vi "Convert Attributes to Name-Value Pairs with Type.vi"(11 "JSON Attributes":string) -> (3 "Name-Value Pairs":T1[](array[typedef]))   [LabVIEW 2015, in "NI_JSON Parsing.lvlib"]
uses:
  NI_JSON Parsing.lvlib
  Name-Value with Type.ctl
  Name Value Pair.ctl
  JSON Type.ctl
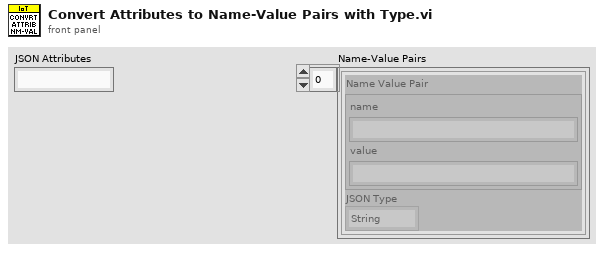
[diagram p1: front panel]
types:
  T1 = typedef "NI_JSON Parsing.lvlib/Name-Value with Type.ctl" = cluster{"Name Value Pair":T2, "JSON Type":T3}
  T2 = typedef "NI_JSON Parsing.lvlib/Name Value Pair.ctl" = cluster{"name":string, "value":string}
  T3 = typedef "NI_JSON Parsing.lvlib/JSON Type.ctl" = enum16{"String", "Numeric", "Boolean"}
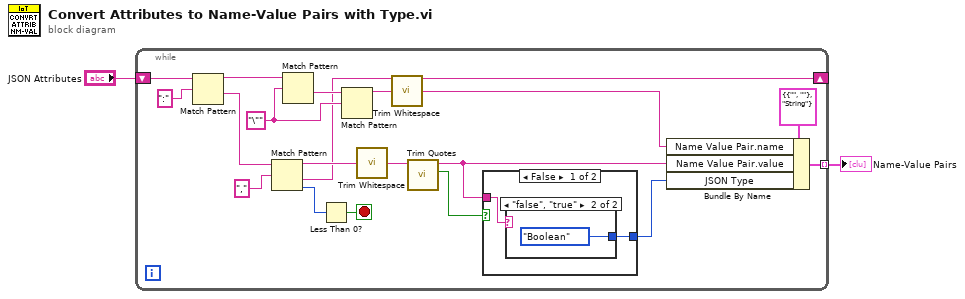
[diagram p0: block diagram]
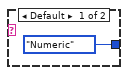
[diagram p2: hidden frame]
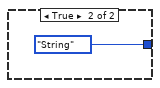
[diagram p3: hidden frame]
diagram:
  n1 = while {
    shift-right: [w10] -> _
    shift-left: "JSON Attributes" -> [w21]
    tunnel: [w8] -> w2 mode=indexing
    stop <- w12 stop-if-true
    w17 = "\"" ("regular expression")
    n2 = Match Pattern(string=w21, regular expression=":") -> (before substring=w19:string, after substring=w15:string)  [unwired: 1 in, 2 out]
    n3 = Match Pattern(string=w15, regular expression=",") -> (before substring=w11:string, after substring=w10:string, offset past match=w13:i32)  [unwired: 1 in, 1 out]
    n4 = Match Pattern(string=w19, regular expression=w17) -> (after substring=w18:string)  [unwired: 1 in, 3 out]
    n5 = Less Than 0?(x=w13) -> (x < 0?=w12:bool)
    n6 = Match Pattern(string=w18, regular expression=w17) -> (before substring=w16:string)  [unwired: 1 in, 3 out]
    n7 = call <vilib>:"Trim Whitespace.vi"("string"=w11) -> ("trimmed string"=w6:string)  [unwired: 1 in]
    n8 = call <vilib>:"Trim Whitespace.vi"("string"=w16) -> ("trimmed string"=w7:string)  [unwired: 1 in]
    n9 = call "Trim Quotes.vi"("String"=w6) -> ("Quotes Trimmed"=w5:bool, "String without Quotes"=w4:string)  [unwired: 9 in]
    n10 = case shown="False" w5 {
      tunnel: w4 -> [w23 _]
      tunnel: [w22 JSON_Type."String" ("JSON Type")] -> w3
      frame False {
        n11 = case shown="\"false\", \"true\"" w23 {
          tunnel: [JSON_Type."Numeric" ("JSON Type") JSON_Type."Boolean" ("JSON Type")] -> w22
          frame Default {
          }
          frame "false", "true" {
          }
        }
      }
      frame True {
      }
    }
    n12 = Bundle By Name(cluster=T1 {"Name Value Pair"={"name"="", "value"=""}, "JSON Type"=enum."String"} ("Name-Value with Type"), "Name Value Pair.name"=w7, "Name Value Pair.value"=w4, "JSON Type"=w3) -> (w8:T1)
  }
  "Name-Value Pairs" <- w2
